vi "meas temp.vi"(7 "DAQ state cluster in":T1={"DAQ state"=enum."Global comm", "device"="", "start (ms)"=0, "error"={"status"=FALSE, "code"=0, "source"=""}, "T cont"={"exec"={"T mode"=enum."Listening to exec", "log"=FALSE, "thermistor"=enum."solo"}, "T status"={"Temp"=0.0}, "utility"={"meas index"=0, "wait (ms)"=0, "therm volt"=0.0, "t T hist"=[]}}} {"T cont"."utility"."therm volt" format="%_6g"; "T cont"."T status"."Temp" format="%_6g"}) -> (8 "DAQ state cluster out":T1={"DAQ state"=enum."Global comm", "device"="", "start (ms)"=0, "error"={"status"=FALSE, "code"=0, "source"=""}, "T cont"={"exec"={"T mode"=enum."Listening to exec", "log"=FALSE, "thermistor"=enum."solo"}, "T status"={"Temp"=0.0}, "utility"={"meas index"=0, "wait (ms)"=0, "therm volt"=0.0, "t T hist"=[]}}} {"T cont"."utility"."therm volt" format="%_6g"; "T cont"."T status"."Temp" format="%_6g"})   [LabVIEW 2019]
doc: "This subVI is one of the states of the DAQ state machine in the thermistoe experiment.\n\nThis state measures the temperature of the thermistor.\n\nIt goes to the wait state next.\n\nPaul K Dixon\nP3600\nCSUSB Physics"
uses:
  typedefs/DAQ T state cluster.ctl
  typedefs/DAQ T state enum.ctl
  typedefs/temp cont cluster.ctl
  typedefs/temp exec cluster.ctl
  typedefs/temp mode enum.ctl
  typedefs/temp indicator.ctl
  typedefs/temp cont utility.ctl
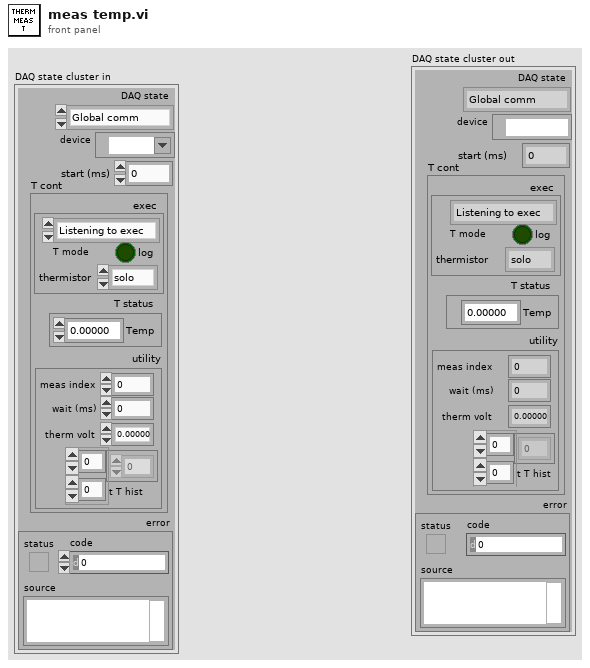
[diagram p1: front panel]
types:
  T1 = typedef "DAQ T state cluster.ctl" = cluster{"DAQ state":T2, "device":tag, "start (ms)":i32, "error":errorcluster, "T cont":T3}
  T2 = typedef "DAQ T state enum.ctl" = enum16{"Global comm", "Meas T ", "Wait", "Exit"}
  T3 = typedef "temp cont cluster.ctl" = cluster{"exec":T4, "T status":T6, "utility":T7}
  T4 = typedef "temp exec cluster.ctl" = cluster{"T mode":T5, "log":bool, "thermistor":enum16{"solo", "bug"}}
  T5 = typedef "temp mode enum.ctl" = enum16{"Setting up", "Listening to exec", "Exit"}
  T6 = typedef "temp indicator.ctl" = cluster{"Temp":dbl}
  T7 = typedef "temp cont utility.ctl" = cluster{"meas index":i32, "wait (ms)":i32, "therm volt":dbl, "t T hist":dbl[][]}
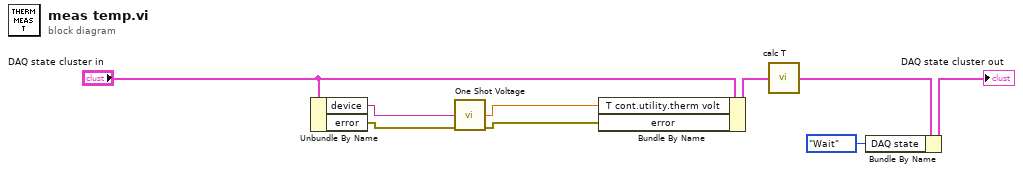
[diagram p0: block diagram]
diagram:
  n1 = Unbundle By Name("DAQ state cluster in") -> ("device"=w4:tag, "error"=w3:errorcluster)
  n2 = call "One Shot Voltage.vi"("device name"=w4, "error in"=w3) -> ("Voltage"=w2:dbl, "error out"=w1:errorcluster)  [unwired: 12 in]
  n3 = Bundle By Name(cluster="DAQ state cluster in", "T cont.utility.therm volt"=w2, "error"=w1) -> (w9:T1)
  n4 = call "calc T.vi"("DAQ state cluster in in"=w9) -> ("DAQ state cluster out"=w8:T1)  [unwired: 14 in]
  n5 = Bundle By Name(cluster=w8, "DAQ state"=DAQ_T_state_enum."Wait") -> (→"DAQ state cluster out":T1)
